vi "Is Done.vi"(8 "Error In":errorcluster, 11 "String In":refnum<class "String.lvclass">) -> (0 "Error Out":errorcluster, 2 "Done":bool, 3 "String Out":refnum<class "String.lvclass">)   [LabVIEW 2017, in "Mustache.lvlib" / "Readers.lvlib" / "String.lvclass"]
uses:
  String.lvclass
  String.lvclass/String.ctl
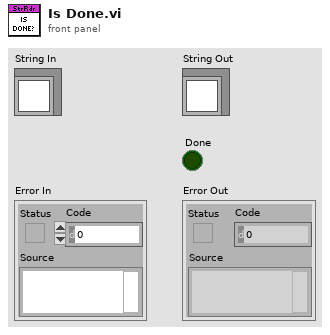
[diagram p1: front panel]
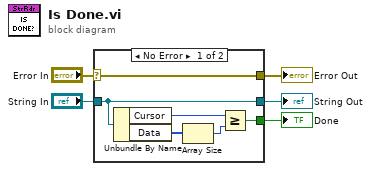
[diagram p0: block diagram]
diagram:
  n1 = case shown="No Error" "Error In" {
    selector: "Error In" -> [w11 w13]
    tunnel: [w11 w13] -> w2
    tunnel: "String In" -> [w10 w12]
    tunnel: [w10 w12] -> w3
    tunnel: [w6 _] -> w1
    frame No Error {
      n2 = Unbundle By Name(w10) -> ("Cursor"=w8:i32, "Data"=w9:u8[])
      n3 = Array Size(array=w9) -> (size(s)=w7:i32)
      n4 = Greater Or Equal?(x=w8, y=w7) -> (x >= y?=w6:bool)
    }
    frame Error {
    }
  }
  "Error Out" <- w2
  "String Out" <- w3
  "Done" <- w1
